vi "start.vi"(8 "error in (no error)":errorcluster, 10 "soundOnly?":bool, 11 "BECHWCBasic in":refnum<class "BECHWCBasic.lvclass">) -> (0 "error out":errorcluster, 2 "started?":bool, 3 "BECHWCBasic out":refnum<class "BECHWCBasic.lvclass">)   [LabVIEW 2011, in "Hardware.lvlib" / "HWControllers.lvlib" / "BECHWCBasic.lvclass"]
doc: "Start running an experiment. I.e. Start all hardware."
uses:
  BECHWCBasic.lvclass
  BECHWCBasic.lvclass/BECHWCBasic.ctl
  HardwareConfiguration/HWConfiguration.lvclass
  Channels/Digital/DigitalOutput.lvclass
  Channels/VoltOutput/AnalogOutput.lvclass
  Tools/Filing/FileNeologist/FileNeologist.lvclass
  HWController.lvclass
  Tools/Filing.lvlib
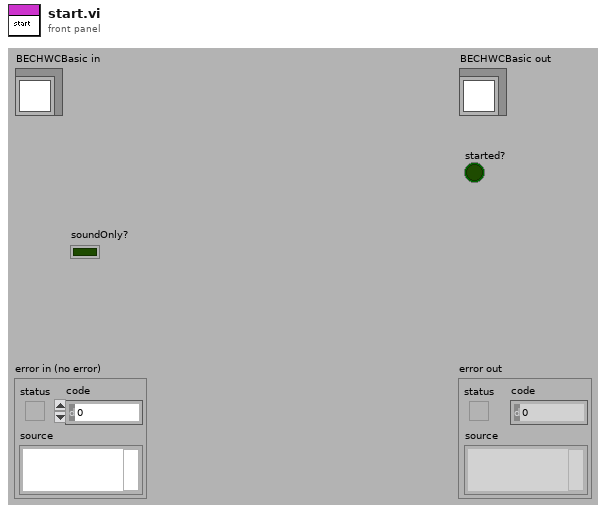
[diagram p1: front panel]
types:
  T1 = enum16{"Ready", "Compiling", "Configured", "Running", "Stopping", "Unresolved Error"}
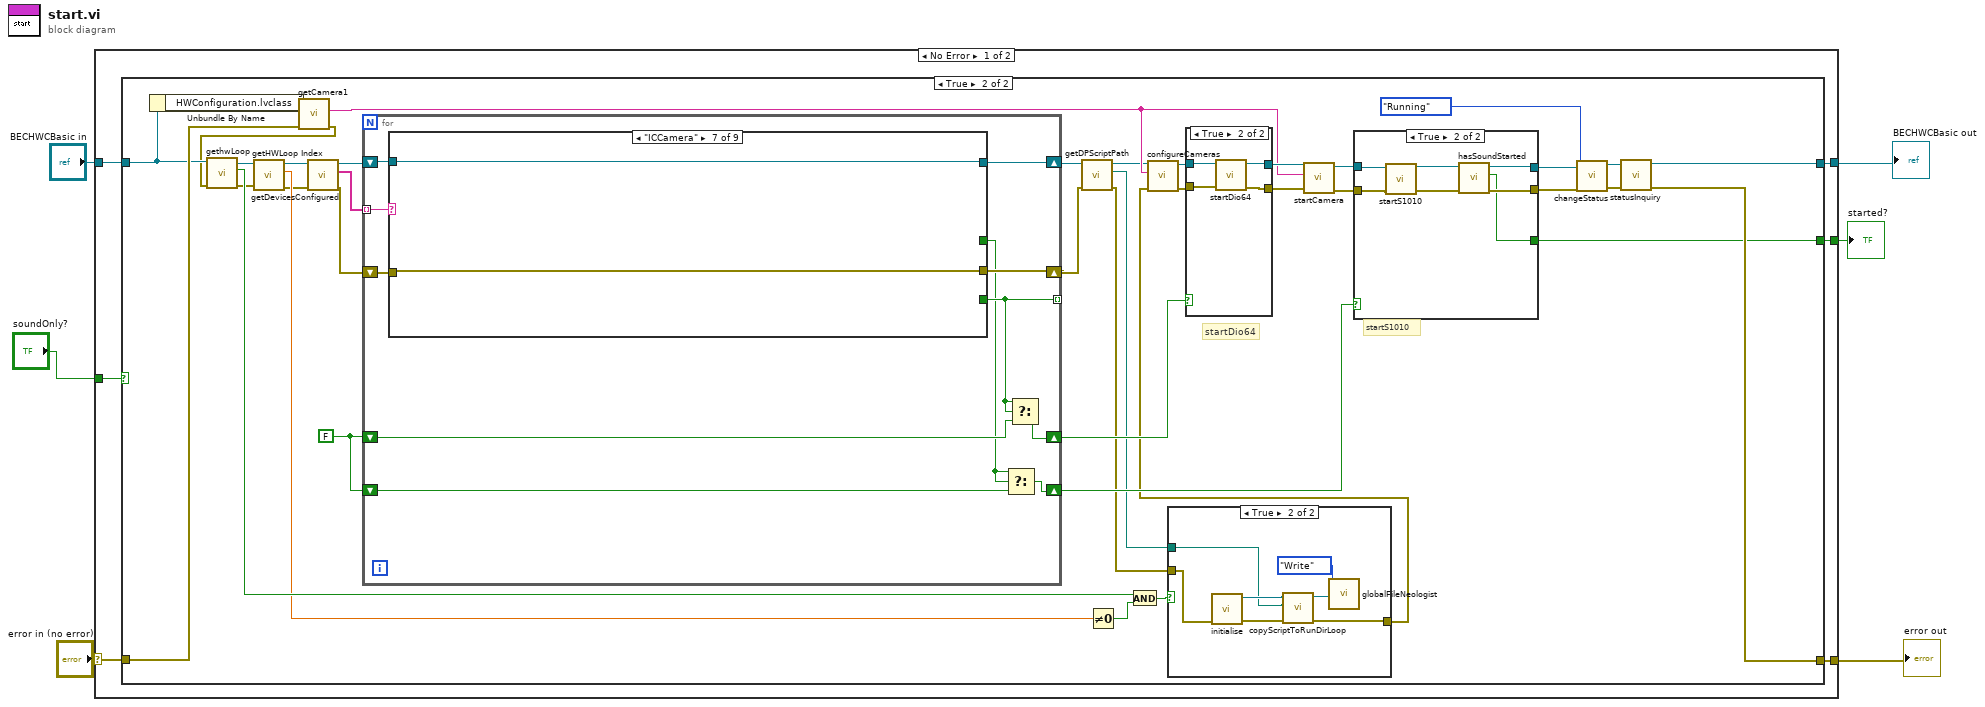
[diagram p0: block diagram]
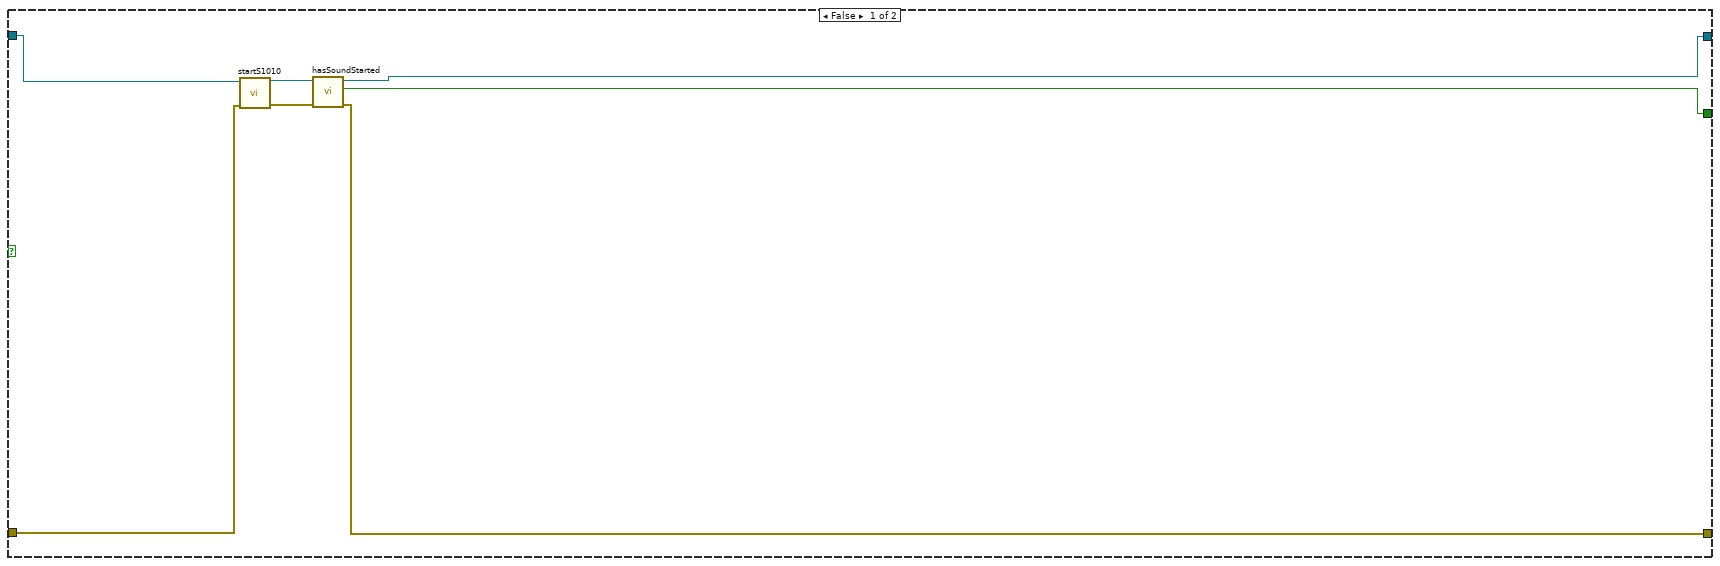
[diagram p2: hidden frame]
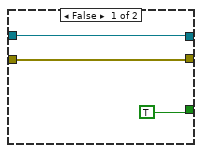
[diagram p4: hidden frame]
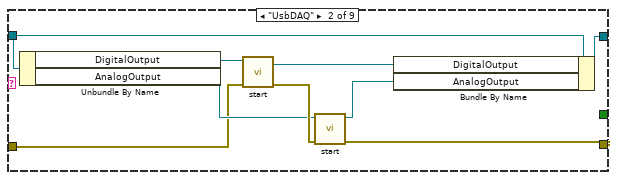
[diagram p7: hidden frame]
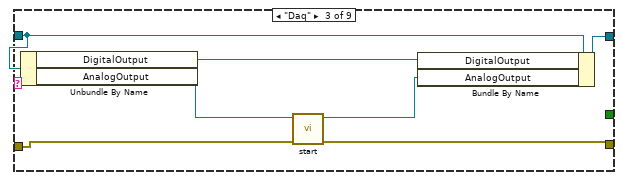
[diagram p8: hidden frame]
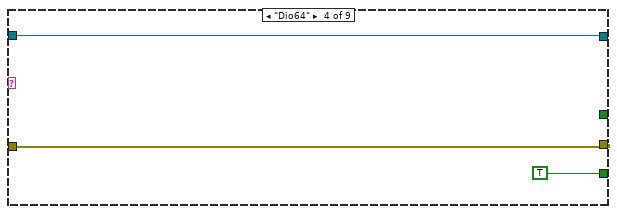
[diagram p9: hidden frame]
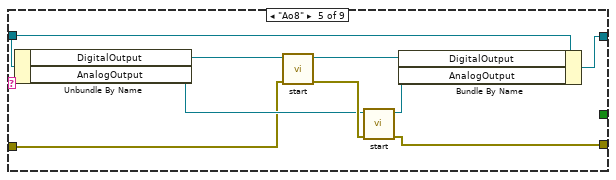
[diagram p10: hidden frame]
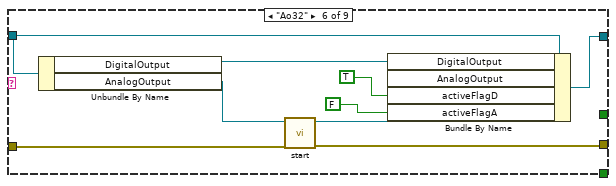
[diagram p11: hidden frame]
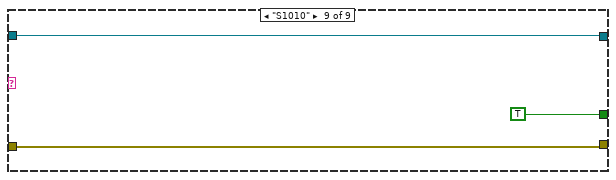
[diagram p13: hidden frame]
diagram:
  n1 = case shown="No Error" "error in (no error)" {
    selector: "error in (no error)" -> [w11 w140]
    tunnel: [w9 w140] -> w5
    tunnel: [w12 w141] -> w3
    tunnel: "BECHWCBasic in" -> [w10 w141]
    tunnel: [w8 _] -> w2
    tunnel: "soundOnly?" -> [w7 _]
    frame No Error {
      n2 = case shown="True" w7 {
        tunnel: [w15 w56] -> w12
        tunnel: w11 -> [w16 w45]
        tunnel: w10 -> [w17 w42]
        tunnel: [w13 w23] -> w9
        tunnel: [w14 w20] -> w8
        frame False {
          n3 = call "startS1010.vi"("error in (no error)"=w16, "BECHWCBasic in"=w17) -> ("error out"=w18:errorcluster, "BECHWCBasic out"=w19:refnum<class "BECHWCBasic.lvclass">)  [unwired: 8 in]
          n4 = call "hasSoundStarted.vi"("error in (no error)"=w18, "BECHWCBasic in"=w19) -> ("error out"=w13:errorcluster, "started?"=w14:bool, "BECHWCBasic out"=w15:refnum<class "BECHWCBasic.lvclass">)  [unwired: 7 in]
        }
        frame True {
          w50 = FALSE
          # "startS1010"
          # "startDio64"
          n5 = Unbundle By Name(w42) -> ("HWConfiguration.lvclass"=w46:refnum<class "HWConfiguration.lvclass">)
          n6 = call-dynamic "getCamera1.vi"("error in (no error)"=w45, "HWConfiguration.lvclass in"=w46) -> ("error out"=w41:errorcluster, "camera1"=w31:string)  [unwired: 7 in, 1 out]
          n7 = call "gethwLoop.vi"("error in (no error)"=w41, "HWController in"=w42) -> ("error out"=w38:errorcluster, "hwLoop?"=w40:bool, "HWController out"=w39:refnum<class "BECHWCBasic.lvclass">)  [unwired: 7 in]
          n8 = call "getHWLoop Index.vi"("error in (no error)"=w38, "HWController in"=w39) -> ("error out"=w33:errorcluster, "HWLoop Index"=w37:dbl, "HWController out"=w34:refnum<class "BECHWCBasic.lvclass">)  [unwired: 7 in]
          n9 = call "getDevicesConfigured.vi"("error in (no error)"=w33, "HWController.lvclass in"=w34) -> ("error out"=w52:errorcluster, "devicesConfigured"=w53:string[], "HWController.lvclass out"=w54:refnum<class "BECHWCBasic.lvclass">)  [unwired: 7 in]
          n10 = for {
            tunnel: w53 -> [w92] mode=indexing
            shift-right: [w90] -> w27
            shift-left: w54 -> [w93]
            shift-right: [w89] -> w25
            shift-left: w52 -> [w91]
            tunnel: [w88] -> _ mode=indexing
            shift-right: [w86] -> w58
            shift-left: w50 -> [w87]
            shift-right: [w83] -> w48
            shift-left: w50 -> [w84]
            n11 = case shown="\"ICCamera\"" w92 {
              tunnel: [w95 w103 w111 w114 w121 w132 w134 w136 w139] -> w90
              tunnel: [w94 w98 w108 w113 w116 w129 w133 w135 w138] -> w89
              tunnel: w93 -> [w95 w104 w110 w114 w122 w131 w134 w136 w139]
              tunnel: w91 -> [w94 w99 w105 w113 w115 w126 w133 w135 w138]
              tunnel: [_ _ _ TRUE _ _ _ _ _] -> w88
              tunnel: [_ _ _ _ _ _ _ _ TRUE] -> w85
              frame "No Hardware", Default {
              }
              frame "UsbDAQ" {
                n12 = Unbundle By Name(w104) -> ("DigitalOutput"=w101:refnum<class "DigitalOutput.lvclass">, "AnalogOutput"=w100:refnum<class "AnalogOutput.lvclass">)
                n13 = call-dynamic "start.vi"("error in (no error)"=w99, "DigitalOutput in"=w101) -> ("error out"=w102:errorcluster, "DigitalOutput out"=w97:refnum<class "DigitalOutput.lvclass">)  [unwired: 8 in]
                n14 = call-dynamic "start.vi"("error in (no error)"=w102, "AnalogOutput in"=w100) -> ("error out"=w98:errorcluster, "AnalogOutput out"=w96:refnum<class "AnalogOutput.lvclass">)  [unwired: 8 in]
                n15 = Bundle By Name(cluster=w104, "DigitalOutput"=w97, "AnalogOutput"=w96) -> (w103:refnum<class "BECHWCBasic.lvclass">)
              }
              frame "Daq" {
                n16 = Unbundle By Name(w110) -> ("DigitalOutput"=w106:refnum<class "DigitalOutput.lvclass">, "AnalogOutput"=w109:refnum<class "AnalogOutput.lvclass">)
                n17 = call-dynamic "start.vi"("error in (no error)"=w105, "AnalogOutput in"=w109) -> ("error out"=w108:errorcluster, "AnalogOutput out"=w107:refnum<class "AnalogOutput.lvclass">)  [unwired: 8 in]
                n18 = Bundle By Name(cluster=w110, "DigitalOutput"=w106, "AnalogOutput"=w107) -> (w111:refnum<class "BECHWCBasic.lvclass">)
              }
              frame "Dio64" {
              }
              frame "Ao8" {
                n19 = Unbundle By Name(w122) -> ("DigitalOutput"=w120:refnum<class "DigitalOutput.lvclass">, "AnalogOutput"=w117:refnum<class "AnalogOutput.lvclass">)
                n20 = call-dynamic "start.vi"("error in (no error)"=w115, "DigitalOutput in"=w120) -> ("error out"=w123:errorcluster, "DigitalOutput out"=w119:refnum<class "DigitalOutput.lvclass">)  [unwired: 8 in]
                n21 = call-dynamic "start.vi"("error in (no error)"=w123, "AnalogOutput in"=w117) -> ("error out"=w116:errorcluster, "AnalogOutput out"=w118:refnum<class "AnalogOutput.lvclass">)  [unwired: 8 in]
                n22 = Bundle By Name(cluster=w122, "DigitalOutput"=w119, "AnalogOutput"=w118) -> (w121:refnum<class "BECHWCBasic.lvclass">)
              }
              frame "Ao32" {
                n23 = Unbundle By Name(w131) -> ("DigitalOutput"=w127:refnum<class "DigitalOutput.lvclass">, "AnalogOutput"=w130:refnum<class "AnalogOutput.lvclass">)
                n24 = call-dynamic "start.vi"("error in (no error)"=w126, "AnalogOutput in"=w130) -> ("error out"=w129:errorcluster, "AnalogOutput out"=w128:refnum<class "AnalogOutput.lvclass">)  [unwired: 8 in]
                n25 = Bundle By Name(cluster=w131, "DigitalOutput"=w127, "AnalogOutput"=w128, "activeFlagD"=TRUE, "activeFlagA"=FALSE) -> (w132:refnum<class "BECHWCBasic.lvclass">)
              }
              frame "ICCamera" {
              }
              frame "AndorIKon" {
              }
              frame "S1010" {
              }
            }
            n26 = Select(t=w85, s=w85, f=w84) -> (s? t:f=w83:bool)
            n27 = Select(t=w88, s=w88, f=w87) -> (s? t:f=w86:bool)
          }
          n28 = call "getDPScriptPath.vi"("error in (no error)"=w25, "HWController in"=w27) -> ("error out"=w22:errorcluster, "DPScriptPath"=w24:path, "HWController out"=w26:refnum<class "BECHWCBasic.lvclass">)  [unwired: 7 in]
          n29 = Not Equal To 0?(x=w37) -> (x != 0?=w36:bool)
          n30 = And(x=w40, y=w36) -> (x .and. y?=w35:bool)
          n31 = case shown="True" w35 {
            tunnel: w22 -> [w59 w65]
            tunnel: w24 -> [_ w61]
            tunnel: [w59 w63] -> w21
            frame False {
            }
            frame True {
              n32 = call "initialise.vi"("error in (no error)"=w65) -> ("error out"=w64:errorcluster, "FileNeologist out"=w62:refnum<class "FileNeologist.lvclass">)  [unwired: 9 in]
              n33 = call-dynamic "copyScriptToRunDirLoop.vi"("error in (no error)"=w64, "Path in"=w61, "FileNeologist in"=w62) -> ("error out"=w63:errorcluster, "FileNeologist out"=w60:refnum<class "FileNeologist.lvclass">)  [unwired: 6 in, 1 out]
              n34 = call "globalFileNeologist.vi"("FileNeologist in"=w60, "Action"=enum16{"Write", "Read"}."Write") -> ()  [unwired: 9 in, 1 out]
            }
          }
          n35 = call "configureCameras.vi"("error in (no error)"=w21, "deviceName"=w31, "BECHWCBasic in"=w26) -> ("error out"=w30:errorcluster, "BECHWCBasic out"=w32:refnum<class "BECHWCBasic.lvclass">)  [unwired: 7 in]
          n36 = case shown="True" w58 {
            tunnel: w32 -> [w78 w82]
            tunnel: [w78 w81] -> w44
            tunnel: w30 -> [w77 w80]
            tunnel: [w77 w79] -> w43
            frame False {
            }
            frame True {
              n37 = call "startDio64.vi"("error in (no error)"=w80, "BECHWCBasic in"=w82) -> ("error out"=w79:errorcluster, "BECHWCBasic out"=w81:refnum<class "BECHWCBasic.lvclass">)  [unwired: 8 in]
            }
          }
          n38 = call "startCamera.vi"("error in (no error)"=w43, "camera"=w31, "BECHWCBasic in"=w44) -> ("error out"=w28:errorcluster, "BECHWCBasic out"=w29:refnum<class "BECHWCBasic.lvclass">)  [unwired: 7 in]
          n39 = case shown="True" w48 {
            tunnel: w29 -> [w69 w76]
            tunnel: [w69 w73] -> w47
            tunnel: w28 -> [w68 w75]
            tunnel: [w68 w72] -> w49
            tunnel: [TRUE w70] -> w20
            frame False {
            }
            frame True {
              n40 = call "startS1010.vi"("error in (no error)"=w75, "BECHWCBasic in"=w76) -> ("error out"=w71:errorcluster, "BECHWCBasic out"=w74:refnum<class "BECHWCBasic.lvclass">)  [unwired: 8 in]
              n41 = call "hasSoundStarted.vi"("error in (no error)"=w71, "BECHWCBasic in"=w74) -> ("error out"=w72:errorcluster, "started?"=w70:bool, "BECHWCBasic out"=w73:refnum<class "BECHWCBasic.lvclass">)  [unwired: 7 in]
            }
          }
          n42 = call "changeStatus.vi"("error in (no error)"=w49, "status"=T1."Running", "HWController in"=w47) -> ("error out"=w55:errorcluster, "HWController out"=w57:refnum<class "BECHWCBasic.lvclass">)  [unwired: 7 in]
          n43 = call-dynamic "statusInquiry.vi"("error in (no error)"=w55, "HWController in"=w57) -> ("error out"=w23:errorcluster, "HWController out"=w56:refnum<class "BECHWCBasic.lvclass">)  [unwired: 8 in]
        }
      }
    }
    frame Error {
    }
  }
  "error out" <- w5
  "BECHWCBasic out" <- w3
  "started?" <- w2
